vi "PRIME Detector Simple Test Program.vi"() -> ()   [LabVIEW 2020]
uses:
  RIMAS Detector Server Config.ctl
  70f956ab-387e-4e3b-bc8c-98fe046a7e37.vi
  PRIME Detector.lvclass
panel:
  out "error out":errorcluster
  out "Responses":string[](array[string])
  out "Status Response":string
  in  "Settings":T1={"Machine"="192.168.121.11", "Password"="", "FITS File Path"="", "Port"=44444, "Header Path"="", "Name"=""}
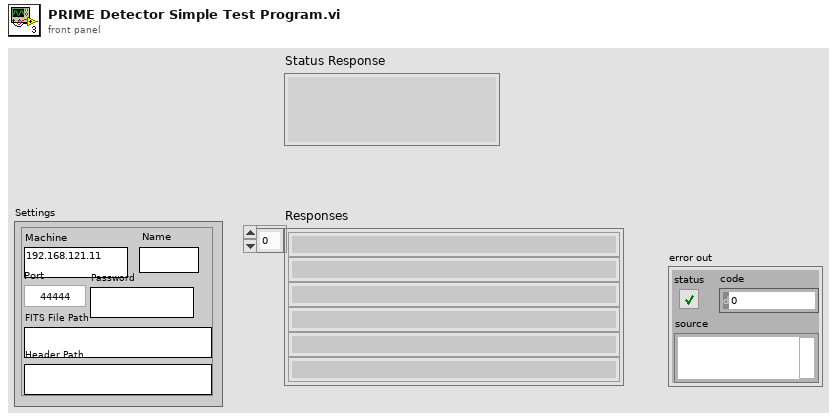
[diagram p1: front panel]
types:
  T1 = typedef "RIMAS Detector Server Config.ctl" = cluster{"Machine":string, "Password":string, "FITS File Path":string, "Port":u16, "Header Path":string, "Name":string}
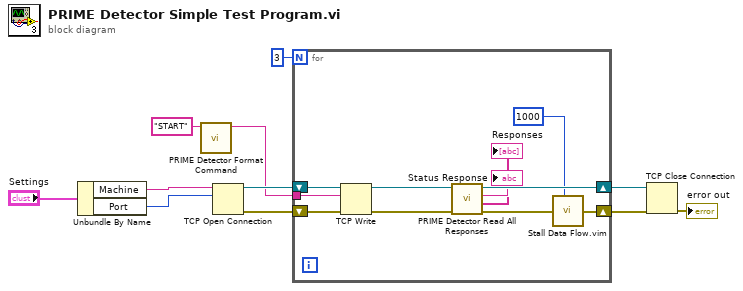
[diagram p0: block diagram]
diagram:
  n1 = Unbundle By Name("Settings") -> ("Machine"=w9:string, "Port"=w10:u16)
  n2 = call "PRIME Detector Format Command.vi"("Command"="START") -> ("TCP String"=w6:string)  [unwired: 10 in]
  n3 = TCP Open Connection(address=w9, remote port or service name=w10) -> (connection ID=w7:refnum<k5>, error out=w5:errorcluster)  [unwired: 3 in]
  n4 = for {
    N: 3 -> [_]
    tunnel: w6 -> [w21]
    shift-right: [w17] -> w4
    shift-left: w7 -> [w22]
    shift-right: [w13] -> w3
    shift-left: w5 -> [w20]
    n5 = TCP Write(connection ID=w22, data in=w21, error in (no error)=w20) -> (connection ID out=w18:refnum<k5>, error out=w19:errorcluster)  [unwired: 1 in, 1 out]
    n6 = call "PRIME Detector Read All Responses.vi"("error in"=w19, "connection ID"=w18) -> ("error out"=w16:errorcluster, "Responses"=→"Responses":string[], "Status Response"=→"Status Response":string, "connection ID out"=w17:refnum<k5>)  [unwired: 6 in]
    n7 = call "Stall Data Flow.vim"("value in"=w16, "milliseconds to wait"=u32 1000) -> ("value out"=w13:errorcluster)  [unwired: 1 out]
  }
  n8 = TCP Close Connection(connection ID=w4, error in (no error)=w3) -> (error out=→"error out":errorcluster)  [unwired: 1 in, 1 out]
